vi "PPG_ABC.set default letter.vi"(0 "i ref in":refnum<vi>, 1 "letter":string, 2 "patternGroup":i32, 3 "ms timeout [ms]":i32=10000, 5 "error in (no error)":errorcluster) -> (14 "i ref out":refnum<vi>, 17 "timed out":bool, 19 "error out":errorcluster)   [LabVIEW 2014, in "PPG_ABC.lvlib"]
doc: "Sets name of the default letter that will be used when executing the next SetTime command.A letter has the format XN, where X denotes a letter between A and Z and N denotes the \"memory index\" (not the number of the time table) starting at 1."
uses:
  PPG_ABC.lvlib
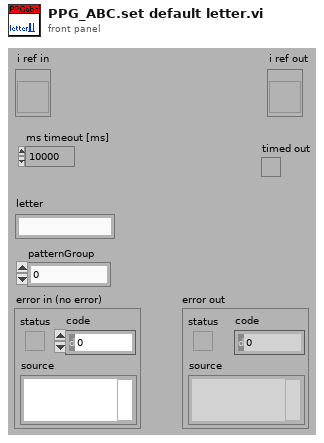
[diagram p1: front panel]
types:
  T1 = typedef "PPG_ABC.lvlib/PPG_ABC.i attribute.ctl" = cluster{"patternGroups":T2[], "defaultLetter":string, "defaultPatternGroup":i32, "PGRunning":T3, "PGRunningID":i32, "pgStarting":T4}
  T2 = typedef "PPG_ABC.lvlib/PPG_ABC.PG_dataType.ctl" = cluster{"PGDevice":string, "rawPatternData":cluster{"triggerCondition":i32, "timeTable":dbl[], "channelTable":string[]}[]}
  T3 = typedef "PPG_ABC.lvlib/PPG_ABC.PG_Running.ctl" = i32
  T4 = typedef "Semaphore RefNum" = refnum<k1>
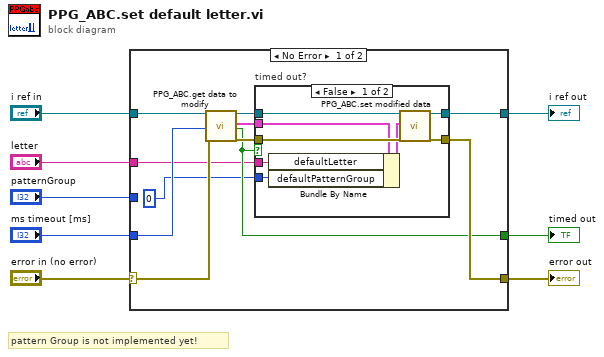
[diagram p0: block diagram]
diagram:
  # "pattern Group is not implemented yet!"
  n1 = case shown="No Error" "error in (no error)" {
    selector: "error in (no error)" -> [w18 w31]
    tunnel: [w14 w31] -> w7
    tunnel: "i ref in" -> [w19 w30]
    tunnel: [w13 w30] -> w5
    tunnel: "letter" -> [w10 _]
    tunnel: [w12 _] -> w3
    tunnel: "ms timeout [ms]" -> [w17 _]
    tunnel: "patternGroup" -> [_ _]
    frame No Error {
      n2 = call "PPG_ABC.get data to modify.vi"("i ref in"=w19, "ms timeout (10000)"=w17, "error in (no error)"=w18) -> ("i ref out"=w16:refnum<vi>, "i attribute"=w11:T1, "timed out"=w12:bool, "error out"=w15:errorcluster)  [unwired: 13 in]
      n3 = case "timed out?" shown="False" w12 {
        tunnel: [w26 w29] -> w13
        tunnel: w16 -> [w27 w29]
        tunnel: w15 -> [w25 w28]
        tunnel: [w24 w28] -> w14
        tunnel: w11 -> [w23 _]
        tunnel: w10 -> [w21 _]
        tunnel: 0 ("patternGroup") -> [w20 _]
        frame False {
          n4 = Bundle By Name(cluster=w23, "defaultLetter"=w21, "defaultPatternGroup"=w20) -> (w22:T1)
          n5 = call "PPG_ABC.set modified data.vi"("i ref in"=w27, "i attribute"=w22, "error in (no error)"=w25) -> ("i ref out"=w26:refnum<vi>, "error out"=w24:errorcluster)  [unwired: 15 in]
        }
        frame True {
        }
      }
    }
    frame Error {
    }
  }
  "error out" <- w7
  "i ref out" <- w5
  "timed out" <- w3
